vi "Camera Test.vi"() -> ()   [LabVIEW 2018]
doc: "This VI implements the framework and scheduler for your robotics program. It should not be necessary to modify the framework. You are expected to add your code to the VIs called from Robot Main - the ones located in the Team Codae folder within the project.\n\nCode is provided As Is. It has not been tested or validated as a product, for use in a deployed application or system, or for use in hazardous environments. You assume all risks for use of the Code and use of the Code is subject to the Sample Code License Terms which can be found at: http://ni.com/samplecodelicense"
uses:
  <vilib>/Utility/file.llb/Write Delimited Spreadsheet (string).vi
  <vilib>/vision/driver/NI_Vision_Acquisition_Software.lvlib
  <resource>/objmgr/imaqdx.rc
panel:
  out "Successful Modes":string[][](table)
  in  "Save Results":bool
  in  "Path":path
  out "Failed Modes":string[][](table)
  out "Camera Name":string
  out "Details":T1(array[cluster])
  out "Progress":i32(slide) scale=0.0..103.0
  out "Image":T2(plugin-control)
  # "This VI implements the framework and scheduler for your robotics program. \nIt should not be necessary to modify the framework. \nYou are expected to add your code to the VIs called from Robot Main, the ones located in the Team Codae folder within the project.\n\nCode is provided As Is and subject to the Sample Code License Terms which can be found at: http://ni.com/samplecodelicense"
  # "Directions:\n1. Plug camera(s) into the controller or computer. Change the target to the controller if necessary.\n2. If you want to save results to a spreadsheet file, set the path to a good location on the target.\n3. Run the VI."
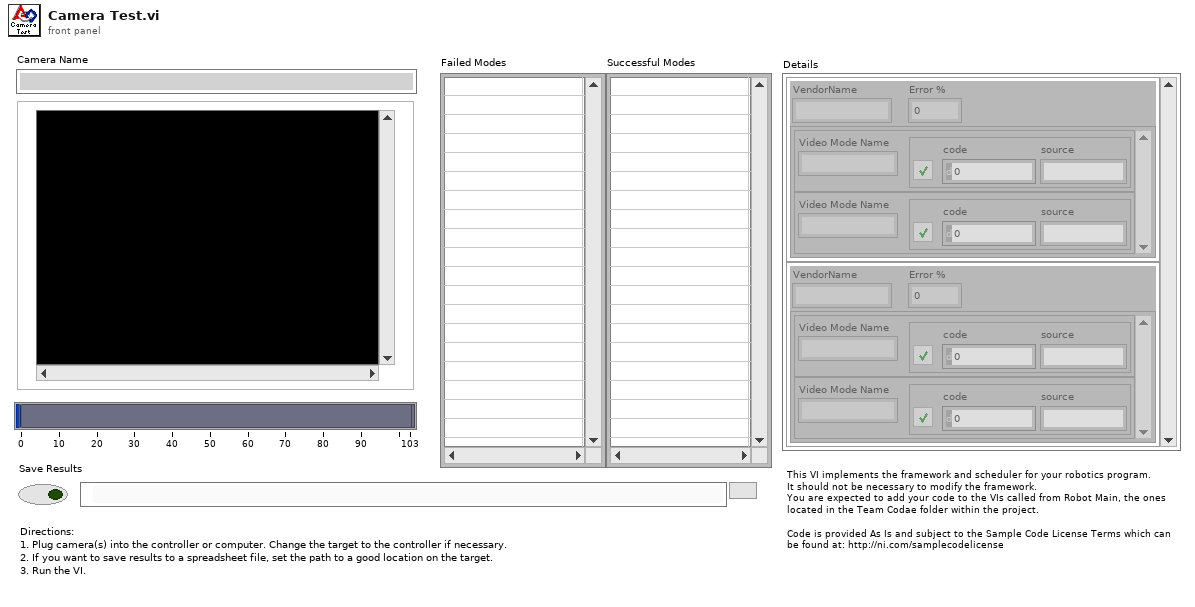
[diagram p1: front panel]
types:
  T1 = cluster{"VendorName":string, cluster{"Video Mode Name":string, "error out":errorcluster}[], "Error %":dbl}[]
  T2 = typedef "IMAQ Image.ctl" = refnum<image>
  T3 = typedef "Image Type" = u32
  T4 = cluster{"Type":u32, "Version":u32, "Flags":u32, "SerialNumberHigh":u32, "SerialNumberLow":u32, "BusType":u32, "InterfaceName":string, "VendorName":string, "ModelName":string, "CameraFileName":string, "CameraAttributeURL":string}[]
  T5 = typedef "IMAQdx.ctl" = refnum<k21>
  T6 = cluster{"Video Mode":u32, "Video Mode Name":string}[]
  T7 = cluster{"Video Mode Name":string, "error out":errorcluster}
  T8 = cluster{"Video Mode Name":string, "error out":errorcluster}[]
  T9 = cluster{"VendorName":string, cluster{"Video Mode Name":string, "error out":errorcluster}[], dbl}
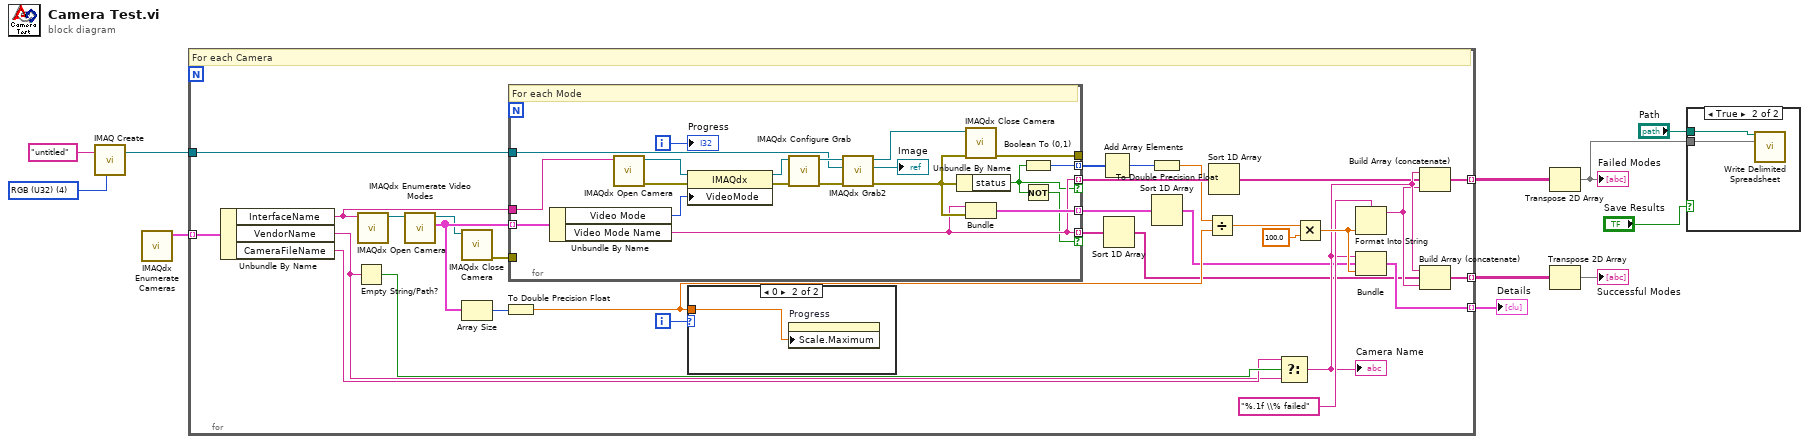
[diagram p0: block diagram]
diagram:
  w8 = T3 4 items=["Grayscale (U8)", "Grayscale (I16)", "Grayscale (SGL)", "Complex (CSG)", "RGB (U32)", "HSL (U32)", "RGB (U64)", "Grayscale (U16)"] ("Image Type")
  n1 = call "IMAQ Create"("Image Name"="untitled", "Image Type"=w8) -> ("New Image"=w9:T2)  [unwired: 3 in, 1 out]
  n2 = call <vilib>:"IMAQdx Enumerate Cameras.vi"() -> ("Camera Information Array"=w11:T4)  [unwired: 10 in, 1 out]
  n3 = for {
    tunnel: w11 -> [w41] mode=indexing
    tunnel: w9 -> [w37]
    tunnel: [w34] -> w7 mode=indexing
    tunnel: [w28] -> w6 mode=indexing
    tunnel: [w18] -> w1 mode=indexing
    i -> [w31]
    # "For each Camera"
    n4 = Unbundle By Name(w41) -> ("InterfaceName"=w36:string, "VendorName"=w21:string, "CameraFileName"=w22:string)
    n5 = Empty String/Path?(string/path=w21) -> (empty?=w23:bool)
    n6 = call <vilib>:"IMAQdx Open Camera.vi"("Session In"=w36) -> ("Session Out"=w42:T5)  [unwired: 9 in, 1 out]
    n7 = call <vilib>:"IMAQdx Enumerate Video Modes.vi"("Session In"=w42) -> ("Video Modes"=w40:T6, "Session Out"=w39:T5)  [unwired: 7 in, 2 out]
    n8 = call <vilib>:"IMAQdx Close Camera.vi"("Session In"=w39) -> ("error out"=w38:errorcluster)  [unwired: 10 in]
    n9 = Array Size(array=w40) -> (size(s)=w30:i32)
    n10 = To Double Precision Float(number=w30) -> (double precision float=w19:dbl)
    n11 = for {
      tunnel: w40 -> [w63] mode=indexing
      tunnel: w38 -> [_]
      tunnel: w37 -> [w56]
      tunnel: [w51] -> w35 mode=indexing
      tunnel: [w50] -> _
      tunnel: w36 -> [w49]
      tunnel: [w47] -> w33 mode=indexing
      tunnel: [w46] -> w29 mode=indexing if=w45
      tunnel: [w46] -> w15 mode=indexing if=w44
      i -> [w58]
      # "For each Mode"
      n12 = Unbundle By Name(w63) -> ("Video Mode"=w62:u32, "Video Mode Name"=w46:string)
      n13 = call <vilib>:"IMAQdx Open Camera.vi"("Session In"=w49) -> ("error out"=w54:errorcluster, "Session Out"=w57:T5)  [unwired: 9 in]
      n14 = property class="IMAQdx"(reference=w57, error in=w54, "VideoMode"=w62) -> (reference out=w61:T5, error out=w53:errorcluster)
      n15 = call <vilib>:"IMAQdx Configure Grab.vi"("error in"=w53, "Session In"=w61) -> ("error out"=w52:errorcluster, "Session Out"=w60:T5)  [unwired: 8 in]
      n16 = call <vilib>:"IMAQdx Grab2.vi"("error in"=w52, "Image In"=w56, "Session In"=w60) -> ("error out"=w48:errorcluster, "Image Out"=→"Image":T2, "Session Out"=w55:T5)  [unwired: 5 in, 1 out]
      n17 = Unbundle By Name(w48) -> ("status"=w45:bool)
      n18 = call <vilib>:"IMAQdx Close Camera.vi"("error in"=w48, "Session In"=w55) -> ("error out"=w50:errorcluster)  [unwired: 9 in]
      n19 = Bundle("Video Mode Name"=w46, "error out"=w48) -> (w51:T7)  [unwired: 1 in]
      n20 = Boolean To (0,1)(Boolean=w45) -> (0, 1=w47:i16)
      n21 = Not(x=w45) -> (.not. x?=w44:bool)
      "Progress" <- w58
    }
    n22 = case shown="0" w31 {
      tunnel: w19 -> [_ w43]
      frame Default {
      }
      frame 0 {
        n23 = property on="Progress" class="Slide (strict)"("Scale.Maximum"=w43) -> ()  [unwired: 2 in, 2 out]
      }
    }
    n24 = Add Array Elements(numeric array=w33) -> (sum=w32:i16)
    n25 = Sort 1D Array(array=w15) -> (sorted array=w14:string[])
    n26 = To Double Precision Float(number=w32) -> (double precision float=w20:dbl)
    n27 = Sort 1D Array(array=w35) -> (sorted array=w12:T8)
    n28 = Divide(x=w20, y=w19) -> (x/y=w27:dbl)
    n29 = Sort 1D Array(array=w29) -> (sorted array=w13:string[])
    n30 = Select(t=w22, s=w23, f=w21) -> (s? t:f=w17:string)
    "Camera Name" <- w17
    n31 = Multiply(x=w27, y=100.0) -> (x*y=w26:dbl)
    n32 = Format Into String(format string="%.1f \\% failed", w26) -> (resulting string=w16:string)  [unwired: 2 in, 1 out]
    n33 = Bundle("VendorName"=w17, w12, w26) -> (w34:T9)  [unwired: 1 in]
    n34 = Build Array (concatenate)(w17, w13, w16) -> (w28:string[])
    n35 = Build Array (concatenate)(w17, w14, w16) -> (w18:string[])
  }
  "Details" <- w7
  n36 = Transpose 2D Array(2D array=w6) -> (transposed array=w3:string[][])
  "Failed Modes" <- w3
  n37 = Transpose 2D Array(2D array=w1) -> (transposed array=→"Successful Modes":string[][])
  n38 = case shown="True" "Save Results" {
    tunnel: "Path" -> [_ w65]
    tunnel: w3 -> [_ w64]
    frame False {
    }
    frame True {
      n39 = call-poly <vilib>:"Write Delimited Spreadsheet.vi"("file path (dialog if empty)"=w65, "2D data"=w64) -> ()  [unwired: 12 in, 2 out]
    }
  }
